vi "BM0211-Image Editing.vi"(8 "error IN":errorcluster, 11 "Running model":string) -> (0 "error out":errorcluster)   [LabVIEW 2015]
uses:
  <vilib>/Utility/miscctls.llb/LVBoundsTypeDef.ctl
  <vilib>/Utility/miscctls.llb/LVPointTypeDef.ctl
panel:
  out "Assembly ST-1":picture
  out "filenames":string[](array[string])
  out "selected path":path
  out "Boolean":bool
  in  "Vertical position":sgl(slide) min=-2000 max=2000 scale=-1000.0..2000.0 scale format="%#.0f"
  in  "Horizontal position":sgl(slide) min=-2000 max=2000 scale=-1000.0..2000.0 scale format="%#.0f"
  in  "Zoom Factor":sgl(slide)=1.0 min=1 max=500 scale=0.0..500.0 scale format="%#.0f"
  out "2D Picture":picture
  in  "Stop Button":bool
  in  "Select Part":u16(ring) items=["P1.JPG", "P2.JPG", "P3.JPG", "P4.JPG", "P5.JPG", "P6.JPG", "P7.JPG", "P8.JPG", "P9.JPG", "P10.JPG", "P11.JPG", "P12.JPG", "P13.JPG", "P14.JPG", "P15.JPG"]
  in  "Save":bool
  in  "Select New":bool
  # "Image Editing"
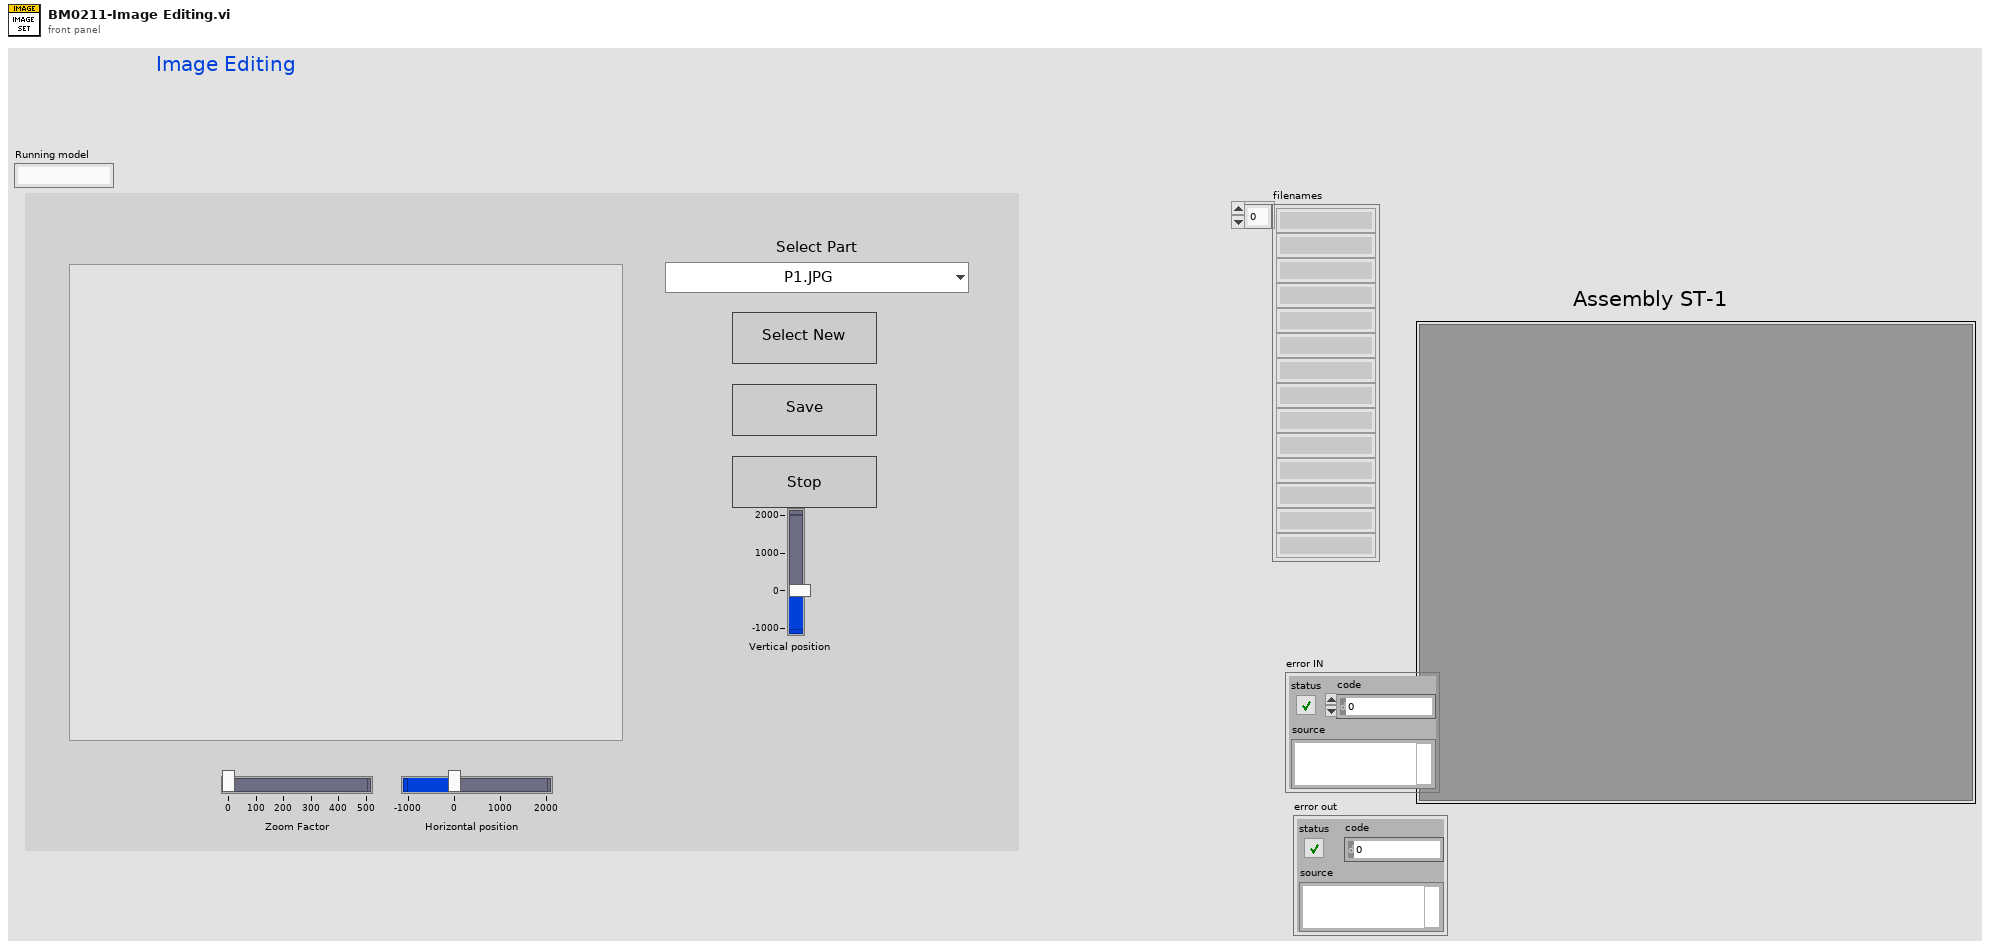
[diagram p1: front panel]
types:
  T1 = typedef "imagedata.ctl" = cluster{"image type":i32, "image depth":i32, "image":u8[], "mask":u8[], "colors":u32[], "Rectangle":cluster{"left":i16, "top":i16, "right":i16, "bottom":i16}}
  T2 = cluster{"Zoom Factor":sgl, "Horizontal position":sgl, "Vertical position":sgl}[]
  T3 = cluster{"Zoom Factor":sgl, "Horizontal position":sgl, "Vertical position":sgl}
  T4 = typedef "LVPointTypeDef.ctl" = cluster{"Horizontal":i16, "Vertical":i16}
  T5 = typedef "LVBoundsTypeDef.ctl" = cluster{"Width":u32, "Height":u32}
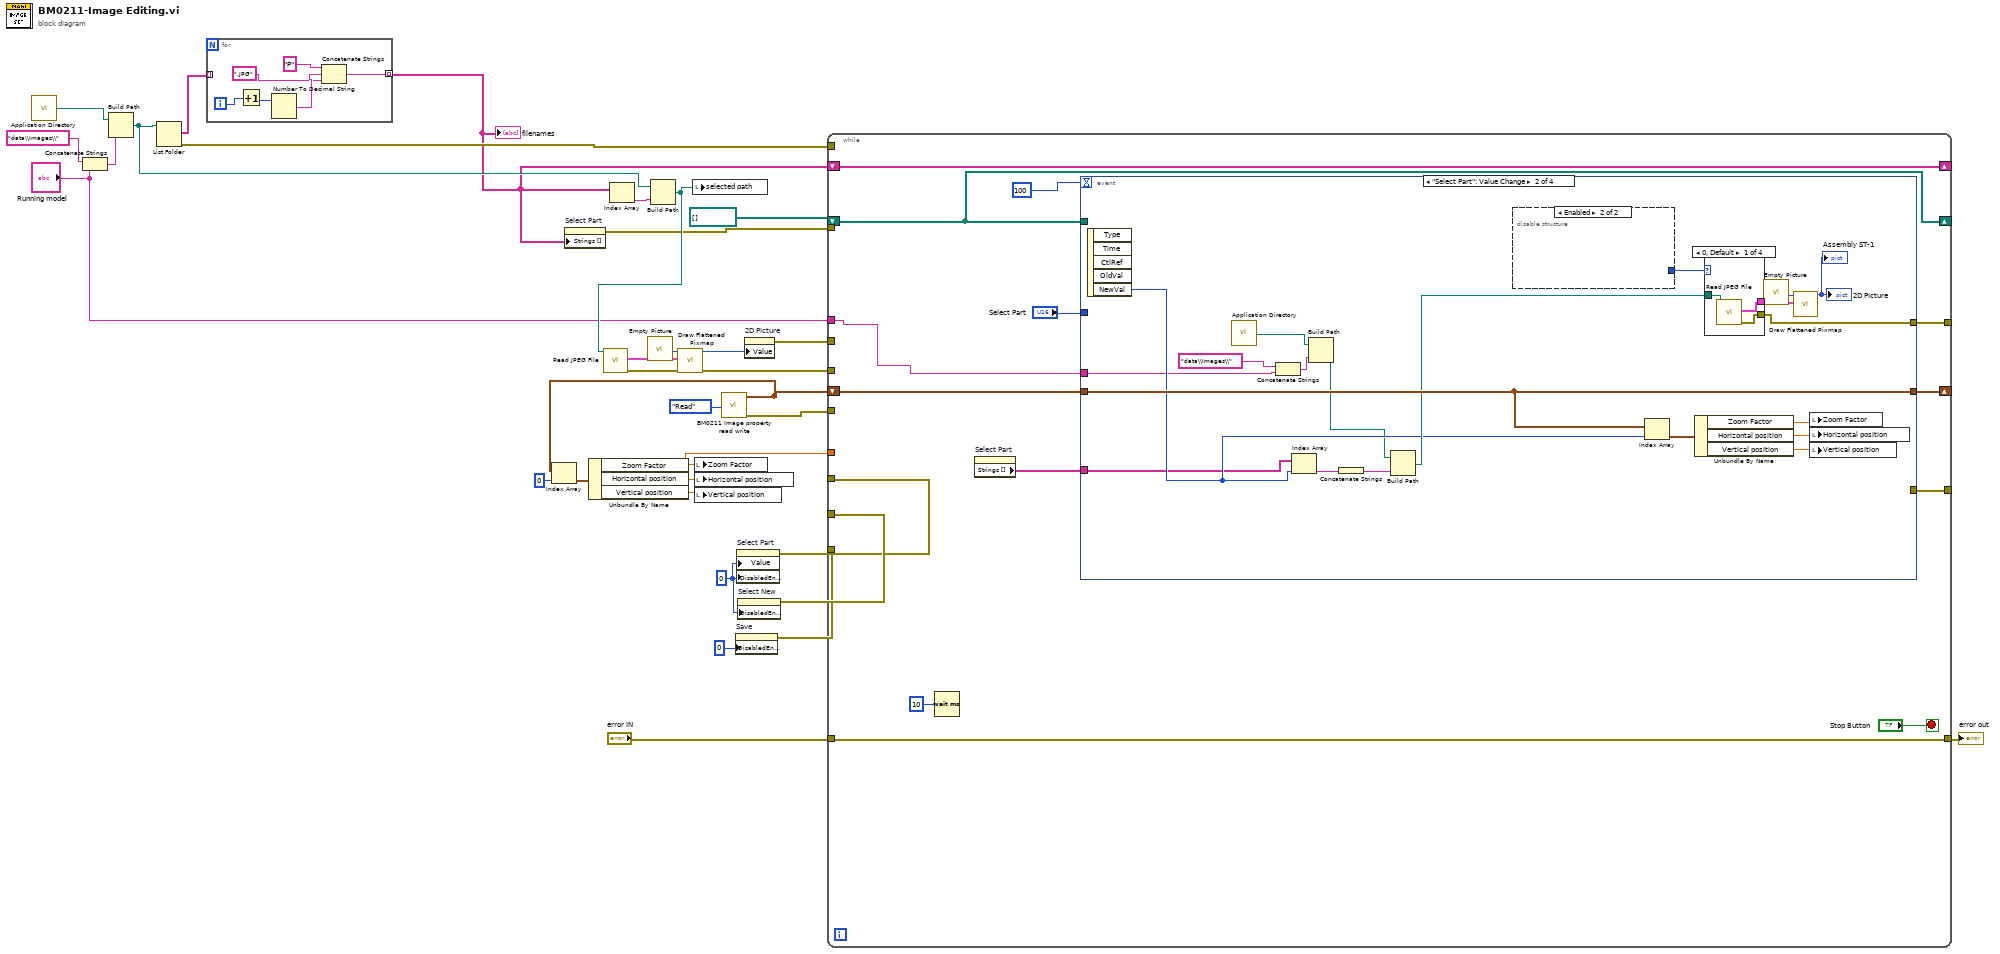
[diagram p0: block diagram]
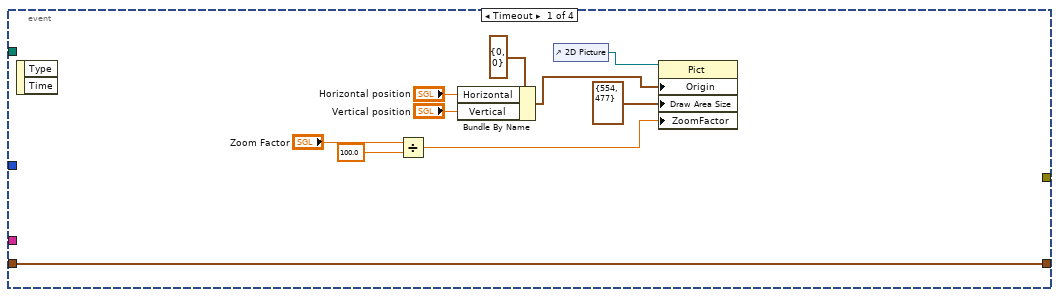
[diagram p2: hidden frame]
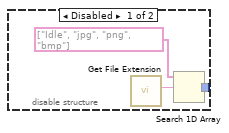
[diagram p3: hidden frame]
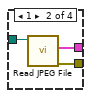
[diagram p4: hidden frame]
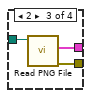
[diagram p5: hidden frame]
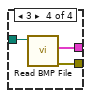
[diagram p6: hidden frame]
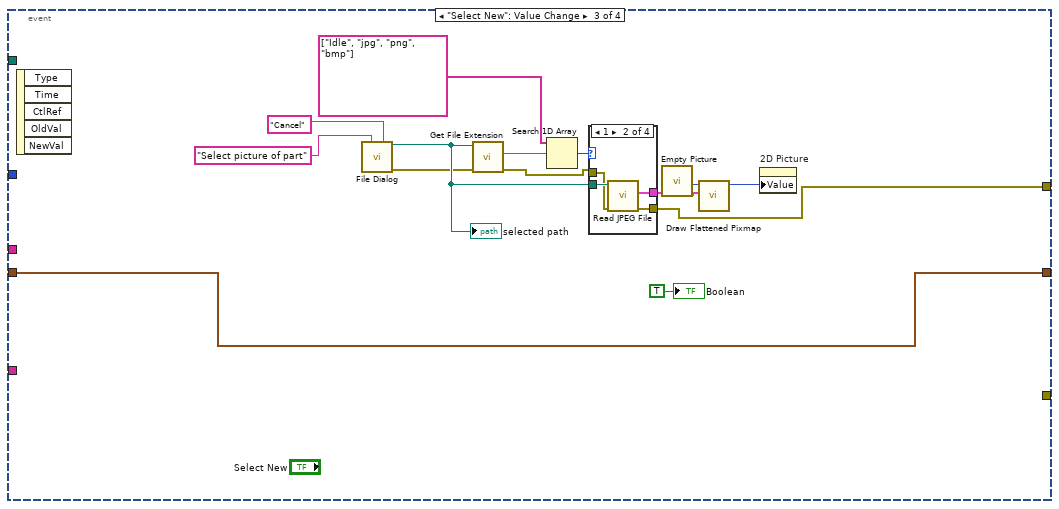
[diagram p7: hidden frame]
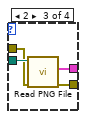
[diagram p9: hidden frame]
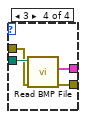
[diagram p10: hidden frame]
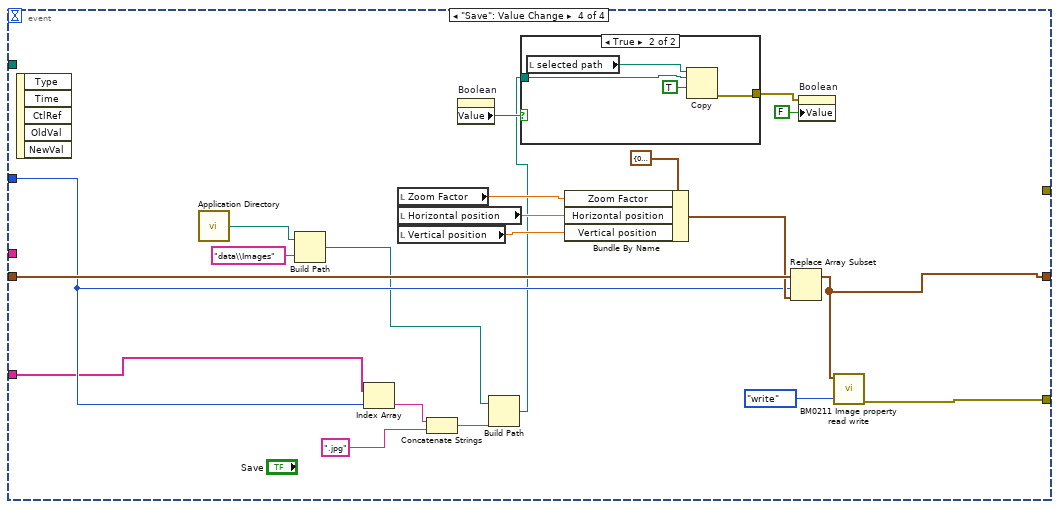
[diagram p11: hidden frame]
diagram:
  w16 = 0
  n1 = call <vilib>:"Application Directory.vi"() -> ("Application Directory"=w10:path)
  n2 = Concatenate Strings("data\\Images\\" ("name or relative path"), "Running model") -> (w2:string)
  n3 = Build Path(base path=w10, name or relative path=w2) -> (appended path=w9:path)
  n4 = List Folder(path=w9) -> (filenames=w5:string[], error out=w15:errorcluster)  [unwired: 3 in, 2 out]
  n5 = for {
    tunnel: w5 -> [_] mode=indexing
    tunnel: [w33] -> w4 mode=indexing
    i -> [w37]
    n6 = Increment(x=w37) -> (x+1=w38:i32)
    n7 = Number To Decimal String(number=w38) -> (decimal integer string=w36:string)  [unwired: 1 in]
    n8 = Concatenate Strings("P" ("string"), w36, ".JPG") -> (w33:string)
  }
  "filenames" <- w4
  n9 = property on="Select Part" class="Ring (strict)"("Strings []"=w4) -> (error out=w8:errorcluster)  [unwired: 2 in, 1 out]
  n10 = Index Array(array=w4) -> (element=w14:string)  [unwired: 1 in]
  n11 = call "Empty Picture"() -> ("empty picture"=w22:picture)
  n12 = Build Path(base path=w9, name or relative path=w14) -> (appended path=w11:path)
  n13 = call <vilib>:"Read JPEG File.vi"("path to JPEG file"=w11) -> ("error out"=w20:errorcluster, "image data"=w21:T1)  [unwired: 8 in, 1 out]
  n14 = call <vilib>:"Draw Flattened Pixmap.vi"("image data"=w21, "picture"=w22) -> ("new picture"=w19:picture)  [unwired: 7 in]
  n15 = local write "selected path"(w11) -> ()
  n16 = call "BM0211 Image property read write.vi"("Read write"=enum16{"write", "Read"}."Read") -> ("error out"=w12:errorcluster, "Out"=w25:T2)  [unwired: 9 in]
  n17 = Index Array(array=w25, index=0) -> (element=w26:T3)
  n18 = Unbundle By Name(w26) -> ("Zoom Factor"=w23:sgl, "Horizontal position"=w27:sgl, "Vertical position"=w28:sgl)
  n19 = local write "Zoom Factor"(w23) -> ()
  n20 = local write "Horizontal position"(w27) -> ()
  n21 = local write "Vertical position"(w28) -> ()
  n22 = property on="Save" class="Bool"("DisabledEnum"=0) -> (error out=w29:errorcluster)  [unwired: 2 in, 1 out]
  n23 = property on="Select Part" class="Ring (strict)"("Value"=w16, "DisabledEnum"=w16) -> (error out=w31:errorcluster)  [unwired: 2 in, 1 out]
  n24 = property on="Select New" class="Bool"("DisabledEnum"=w16) -> (error out=w32:errorcluster)  [unwired: 2 in, 1 out]
  n25 = property on="2D Picture" class="Pict"("Value"=w19) -> (error out=w18:errorcluster)  [unwired: 2 in, 1 out]
  n26 = while {
    shift-right: [w49] -> _
    shift-left: path[] [] ("Array") -> [w49]
    tunnel: [w48] -> _
    shift-right: [w45] -> _
    shift-left: w25 -> [w47]
    tunnel: w32 -> [_]
    tunnel: w31 -> [_]
    tunnel: w29 -> [_]
    tunnel: w23 -> [_]
    tunnel: w20 -> [_]
    tunnel: w18 -> [_]
    tunnel: w15 -> [_]
    shift-right: [w43] -> _
    shift-left: w4 -> [w43]
    tunnel: w12 -> [_]
    tunnel: [w42] -> _
    tunnel: w8 -> [_]
    tunnel: "error IN" -> [w40]
    tunnel: [w40] -> w6
    tunnel: "Running model" -> [w39]
    stop <- "Stop Button" stop-if-true
    n27 = Wait (ms)(milliseconds to wait=u32 10) -> ()  [unwired: 1 out]
    n28 = property on="Select Part" class="Ring (strict)"() -> ("Strings []"=w41:string[])  [unwired: 2 in, 2 out]
    n29 = event shown="[1] \"Select Part\": Value Change" {
      selector: _ -> [_ _ _ _]
      dyn-events: _ -> [_ _ _ _]
      timeout: 100 -> [_ _ _ _]
      tunnel: w49 -> [_ _ _ _]
      tunnel: [_ w80 w99 _] -> w48
      tunnel: w47 -> [w52 w77 w97 w137]
      tunnel: "Select Part" -> [_ _ _ w134]
      tunnel: [w52 w77 w97 w129] -> w45
      tunnel: [_ _ _ w132] -> w42
      tunnel: w41 -> [_ w66 _ w125]
      tunnel: w39 -> [_ w63 _ _]
      event Timeout {
        n30 = event-data() -> ()  [unwired: 1 in, 2 out]
        n31 = Divide(x="Zoom Factor", y=sgl 100.0 ("x")) -> (x/y=w58:sgl)
        n32 = Bundle By Name(cluster=T4 {"Horizontal"=0, "Vertical"=0} ("Origin"), "Horizontal"="Horizontal position", "Vertical"="Vertical position") -> (w54:T4)
        n33 = control-ref of="2D Picture"() -> (w59:refnum<vi>)
        n34 = property class="Pict"(reference=w59, "Origin"=w54, "Draw Area Size"=T5 {"Width"=554, "Height"=477}, "ZoomFactor"=w58) -> ()  [unwired: 1 in, 2 out]
      }
      event "Select Part": Value Change {
        n35 = event-data() -> ("NewVal"=w69:u16)  [unwired: 1 in, 4 out]
        n36 = call <vilib>:"Application Directory.vi"() -> ("Application Directory"=w68:path)
        n37 = Concatenate Strings("data\\Images\\" ("name or relative path"), w63) -> (w62:string)
        n38 = Index Array(array=w66, index=w69) -> (element=w72:string)
        n39 = Build Path(base path=w68, name or relative path=w62) -> (appended path=w67:path)
        n40 = Concatenate Strings(w72) -> (w70:string)
        n41 = Build Path(base path=w67, name or relative path=w70) -> (appended path=w71:path)
        n42 = disable-structure shown="Enabled" {
          disable-tunnel: [w82 _] -> w79
          frame Disabled {
            n43 = call <vilib>:"Get File Extension.vi"() -> ("lowercase file extension"=w83:string)  [unwired: 7 in, 4 out]
            n44 = Search 1D Array(1D array=string[] ["Idle", "jpg", "png", "bmp"] ("Strings []"), element=w83) -> (index of element=w82:i32)  [unwired: 1 in]
          }
          frame Enabled {
          }
        }
        n45 = Index Array(array=w77, index=w69) -> (element=w76:T3)
        n46 = Unbundle By Name(w76) -> ("Zoom Factor"=w75:sgl, "Horizontal position"=w74:sgl, "Vertical position"=w73:sgl)
        n47 = case shown="0, Default" w79 {
          tunnel: [w86 w90 w92 w95] -> w78
          tunnel: [w85 w89 w91 w96] -> w80
          tunnel: w71 -> [w87 w88 w93 w94]
          frame 0, Default {
            n48 = call <vilib>:"Read JPEG File.vi"("path to JPEG file"=w87) -> ("error out"=w85:errorcluster, "image data"=w86:T1)  [unwired: 8 in, 1 out]
          }
          frame 1 {
            n49 = call <vilib>:"Read JPEG File.vi"("path to JPEG file"=w88) -> ("error out"=w89:errorcluster, "image data"=w90:T1)  [unwired: 8 in, 1 out]
          }
          frame 2 {
            n50 = call <vilib>:"Read PNG File.vi"("path to PNG file"=w93) -> ("error out"=w91:errorcluster, "image data"=w92:T1)  [unwired: 8 in, 1 out]
          }
          frame 3 {
            n51 = call <vilib>:"Read BMP File.vi"("path to BMP file"=w94) -> ("error out"=w96:errorcluster, "image data"=w95:T1)  [unwired: 8 in, 1 out]
          }
        }
        n52 = call "Empty Picture"() -> ("empty picture"=w81:picture)
        n53 = call <vilib>:"Draw Flattened Pixmap.vi"("image data"=w78, "picture"=w81) -> ("new picture"=→"2D Picture" →"Assembly ST-1":picture)  [unwired: 7 in]
        n54 = local write "Zoom Factor"(w75) -> ()
        n55 = local write "Horizontal position"(w74) -> ()
        n56 = local write "Vertical position"(w73) -> ()
      }
      event "Select New": Value Change {
        n57 = event-data() -> ()  [unwired: 1 in, 5 out]
        n58 = call "File Dialog"("prompt"="Select picture of part", "button label"="Cancel") -> ("selected path"=w102:path, "error out"=w101:errorcluster)  [unwired: 10 in, 2 out]
        "selected path" <- w102
        n59 = call <vilib>:"Get File Extension.vi"("error in (no error)"=w101, "file"=w102) -> ("error out"=w106:errorcluster, "lowercase file extension"=w108:string)  [unwired: 5 in, 3 out]
        n60 = Search 1D Array(1D array=string[] ["Idle", "jpg", "png", "bmp"] ("Strings []"), element=w108) -> (index of element=w107:i32)  [unwired: 1 in]
        n61 = case shown="1" w107 {
          tunnel: [_ w115 w119 w122] -> w100
          tunnel: [w111 w114 w118 w123] -> w99
          tunnel: w106 -> [w111 w112 w116 w120]
          tunnel: w102 -> [_ w113 w117 w121]
          frame 0, Default {
          }
          frame 1 {
            n62 = call <vilib>:"Read JPEG File.vi"("error in (no error)"=w112, "path to JPEG file"=w113) -> ("error out"=w114:errorcluster, "image data"=w115:T1)  [unwired: 7 in, 1 out]
          }
          frame 2 {
            n63 = call <vilib>:"Read PNG File.vi"("error in (no error)"=w116, "path to PNG file"=w117) -> ("error out"=w118:errorcluster, "image data"=w119:T1)  [unwired: 7 in, 1 out]
          }
          frame 3 {
            n64 = call <vilib>:"Read BMP File.vi"("error in (no error)"=w120, "path to BMP file"=w121) -> ("error out"=w123:errorcluster, "image data"=w122:T1)  [unwired: 7 in, 1 out]
          }
        }
        n65 = call "Empty Picture"() -> ("empty picture"=w110:picture)
        n66 = call <vilib>:"Draw Flattened Pixmap.vi"("image data"=w100, "picture"=w110) -> ("new picture"=w105:picture)  [unwired: 7 in]
        n67 = property on="2D Picture" class="Pict"("Value"=w105) -> ()  [unwired: 2 in, 2 out]
        "Boolean" <- TRUE
      }
      event "Save": Value Change {
        n68 = event-data() -> ()  [unwired: 1 in, 5 out]
        n69 = call <vilib>:"Application Directory.vi"() -> ("Application Directory"=w128:path)
        n70 = Build Path(base path=w128, name or relative path="data\\Images") -> (appended path=w126:path)
        n71 = Index Array(array=w125, index=w134) -> (element=w124:string)
        n72 = local read "Zoom Factor"() -> (w141:sgl)
        n73 = local read "Horizontal position"() -> (w140:sgl)
        n74 = local read "Vertical position"() -> (w139:sgl)
        n75 = Concatenate Strings(w124, ".jpg" ("string")) -> (w131:string)
        n76 = property on="Boolean" class="Bool (strict)"() -> ("Value"=w144:bool)  [unwired: 2 in, 2 out]
        n77 = Build Path(base path=w126, name or relative path=w131) -> (appended path=w133:path)
        n78 = case shown="True" w144 {
          tunnel: w133 -> [_ w145]
          tunnel: [_ w148] -> w142
          frame False {
          }
          frame True {
            n79 = local read "selected path"() -> (w147:path)
            n80 = Copy(9:TRUE ("overwrite (F)"), 10:w145, 11:w147) -> (0:w148:errorcluster)  [unwired: 2 in, 2 out]
          }
        }
        n81 = Bundle By Name(cluster=T3 {"Zoom Factor"=0.0, "Horizontal position"=0.0, "Vertical position"=0.0} ("element"), "Zoom Factor"=w141, "Horizontal position"=w140, "Vertical position"=w139) -> (w136:T3)
        n82 = Replace Array Subset(array=w137, new element=w136, index=w134) -> (w129:T2)
        n83 = property on="Boolean" class="Bool (strict)"(error in=w142, "Value"=FALSE ("Boolean")) -> ()  [unwired: 1 in, 2 out]
        n84 = call "BM0211 Image property read write.vi"("Read write"=enum16{"write", "Read"}."write", "IN"=w129) -> ("error out"=w132:errorcluster)  [unwired: 8 in, 1 out]
      }
    }
  }
  "error out" <- w6
